vi "oduzmi1kapsulu.vi"(8 "error in":errorcluster, 10 "Izbor kafe":T1, 11 "Broj kafa ulaz":T2) -> (0 "error out":errorcluster, 3 "Broj kafa izlaz":T2)   [LabVIEW 2019]
doc: "Oduzimanje jedne kapsule odgovarajuće vrste kafe, ako je to moguće. Ako ulaz nije validan samo se propagira rezultat.\nUlazi su:\n1. Cluster sa 3 broja - broj dostupnih kapsula za 3 vrste kafe\n2. promenljiva enum type def-a IzborKafa\n3. vrednost greške na ulazu\nIzlazi su:\n1. Cluster sa 3 broja - broj dostupnih kapsula nakon ovoga\n2. vrednost greške na izlazu"
uses:
  vrste_kafe.ctl
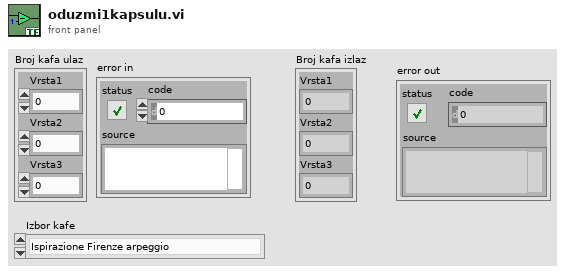
[diagram p1: front panel]
types:
  T1 = typedef "vrste_kafe.ctl" = enum16{"Ispirazione Firenze arpeggio", "Barista Corto", "Ispirazione Napoli"}
  T2 = cluster{"Vrsta1":dbl, "Vrsta2":dbl, "Vrsta3":dbl}
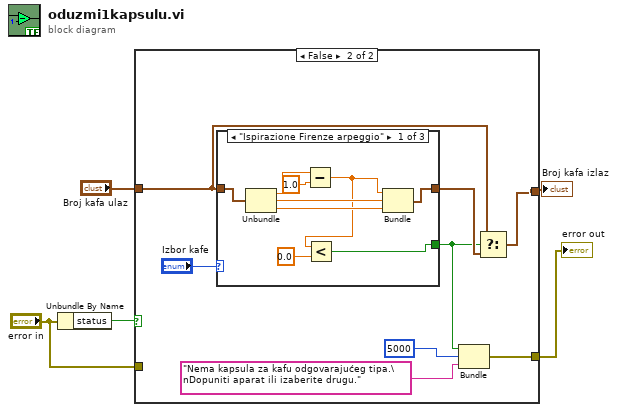
[diagram p0: block diagram]
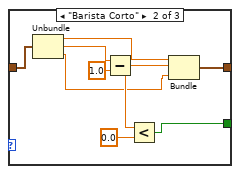
[diagram p3: hidden frame]
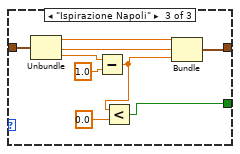
[diagram p4: hidden frame]
diagram:
  n1 = Unbundle By Name("error in") -> ("status"=w3:bool)
  n2 = case shown="False" w3 {
    tunnel: [w7 w14] -> w5
    tunnel: "Broj kafa ulaz" -> [w7 w12]
    tunnel: "error in" -> [w6 _]
    tunnel: [w6 w11] -> w1
    frame True {
    }
    frame False {
      n3 = case shown="\"Ispirazione Firenze arpeggio\"" "Izbor kafe" {
        tunnel: w12 -> [w24 w31 w39]
        tunnel: [w21 w30 w36] -> w13
        tunnel: [w16 w25 w34] -> w10
        frame "Ispirazione Firenze arpeggio" {
          n4 = Unbundle(w24) -> ("Vrsta1"=w22:dbl, "Vrsta2"=w20:dbl, "Vrsta3"=w19:dbl)
          n5 = Subtract(x=w22, y=1.0) -> (x-y=w17:dbl)
          n6 = Less?(x=w17, y=0.0) -> (x < y?=w16:bool)
          n7 = Bundle(w17, "Vrsta2"=w20, "Vrsta3"=w19) -> (w21:cluster{dbl, "Vrsta2":dbl, "Vrsta3":dbl})  [unwired: 1 in]
        }
        frame "Barista Corto" {
          n8 = Unbundle(w31) -> ("Vrsta1"=w27:dbl, "Vrsta2"=w29:dbl, "Vrsta3"=w26:dbl)
          n9 = Subtract(x=w29, y=1.0) -> (x-y=w28:dbl)
          n10 = Less?(x=w28, y=0.0) -> (x < y?=w25:bool)
          n11 = Bundle("Vrsta1"=w27, w28, "Vrsta3"=w26) -> (w30:cluster{"Vrsta1":dbl, dbl, "Vrsta3":dbl})  [unwired: 1 in]
        }
        frame "Ispirazione Napoli" {
          n12 = Unbundle(w39) -> ("Vrsta1"=w37:dbl, "Vrsta2"=w42:dbl, "Vrsta3"=w38:dbl)
          n13 = Subtract(x=w38, y=1.0) -> (x-y=w35:dbl)
          n14 = Less?(x=w35, y=0.0) -> (x < y?=w34:bool)
          n15 = Bundle("Vrsta1"=w37, "Vrsta2"=w42, w35) -> (w36:cluster{"Vrsta1":dbl, "Vrsta2":dbl, dbl})  [unwired: 1 in]
        }
      }
      n16 = Bundle(w10, 5000, "Nema kapsula za kafu odgovarajućeg tipa.\nDopuniti aparat ili izaberite drugu.") -> (w11:errorcluster)  [unwired: 1 in]
      n17 = Select(t=w12, s=w10, f=w13) -> (s? t:f=w14:T2)
    }
  }
  "Broj kafa izlaz" <- w5
  "error out" <- w1
